vi "Delete Event.vi"(8 "error in (no error)":errorcluster, 10 "event id":u32, 11 "eLab in":refnum<class "PL eLabFTW Client.lvclass">) -> (0 "error out":errorcluster, 3 "eLab out":refnum<class "PL eLabFTW Client.lvclass">)   [LabVIEW 2015, in "PL eLabFTW Client.lvclass"]
doc: "Deletes event with the specified id."
uses:
  PL eLabFTW Client.lvclass
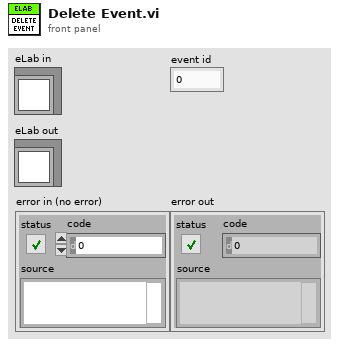
[diagram p1: front panel]
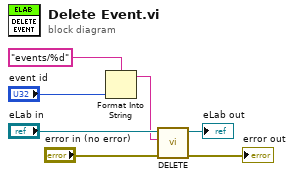
[diagram p0: block diagram]
diagram:
  n1 = Format Into String(format string="events/%d", "event id") -> (resulting string=w3:string)  [unwired: 2 in, 1 out]
  n2 = call "DELETE.vi"("error in (no error)"="error in (no error)", "relative URL"=w3, "eLab in"="eLab in") -> ("error out"=→"error out":errorcluster, "eLab out"=→"eLab out":refnum<class "PL eLabFTW Client.lvclass">)  [unwired: 6 in, 1 out]
